vi "C.vi"(3 "t":dbl, 4 "n^2":dbl, 5 "Promien krzywizny południka [v]":dbl, 6 "fi[rad]":dbl) -> (0 "C":dbl)   [LabVIEW 2015, in "Biblioteka moduł map v3.lvlib" / "Konwersja wsp.lvlib" / "UTM.lvlib" / "Konwersja na UTM.lvlib"]
doc: "Współczynnik wzoru na konwersję na UTM."
uses:
  Konwersja na UTM.lvlib
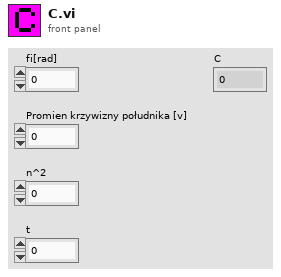
[diagram p1: front panel]
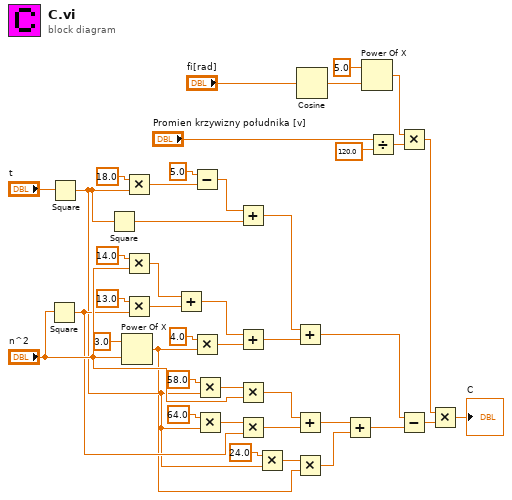
[diagram p0: block diagram]
diagram:
  n1 = Square(x="n^2") -> (x^2=w10:dbl)
  n2 = Square(x="t") -> (x^2=w5:dbl)
  n3 = Square(x=w5) -> (x^2=w28:dbl)
  n4 = Power Of X(1:"n^2", 2:3.0 ("y")) -> (0:w4:dbl)
  n5 = Multiply(x=18.0, y=w5) -> (x*y=w30:dbl)
  n6 = Multiply(x=14.0, y="n^2") -> (x*y=w26:dbl)
  n7 = Multiply(x=13.0, y=w10) -> (x*y=w24:dbl)
  n8 = Add(x=w26, y=w24) -> (x+y=w23:dbl)
  n9 = Subtract(x=5.0, y=w30) -> (x-y=w29:dbl)
  n10 = Multiply(x=4.0, y=w4) -> (x*y=w21:dbl)
  n11 = Multiply(x=58.0, y=w5) -> (x*y=w15:dbl)
  n12 = Multiply(x=64.0, y=w5) -> (x*y=w11:dbl)
  n13 = Add(x=w29, y=w28) -> (x+y=w19:dbl)
  n14 = Add(x=w23, y=w21) -> (x+y=w18:dbl)
  n15 = Multiply(x=w15, y="n^2") -> (x*y=w13:dbl)
  n16 = Multiply(x=w11, y=w10) -> (x*y=w9:dbl)
  n17 = Multiply(x=24.0, y=w5) -> (x*y=w8:dbl)
  n18 = Add(x=w19, y=w18) -> (x+y=w17:dbl)
  n19 = Add(x=w13, y=w9) -> (x+y=w3:dbl)
  n20 = Multiply(x=w8, y=w4) -> (x*y=w6:dbl)
  n21 = Cosine(x="fi[rad]") -> (cos(x)=w37:dbl)
  n22 = Add(x=w3, y=w6) -> (x+y=w2:dbl)
  n23 = Power Of X(1:w37, 2:5.0 ("y")) -> (0:w39:dbl)
  n24 = Divide(x="Promien krzywizny południka [v]", y=120.0) -> (x/y=w40:dbl)
  n25 = Multiply(x=w39, y=w40) -> (x*y=w41:dbl)
  n26 = Subtract(x=w17, y=w2) -> (x-y=w1:dbl)
  n27 = Multiply(x=w41, y=w1) -> (x*y=→"C":dbl)
